vi "MRC Ds Comms Control Set Joystick Outputs.vi"(8 "error in (no error)":errorcluster, 10 "outputs":T1, 11 "stickIndex":i32) -> (0 "error out":errorcluster)   [LabVIEW 2026, in "MrcLib.lvlib"]
doc: "MRC_Status MRC_CALLCONV MRC_DsCommsControl_SetJoystickOutputs(int32_t stickIndex, const struct MRC_JoystickOutputs* outputs);"
uses:
  MrcLib.lvlib
  MrcLib.dll
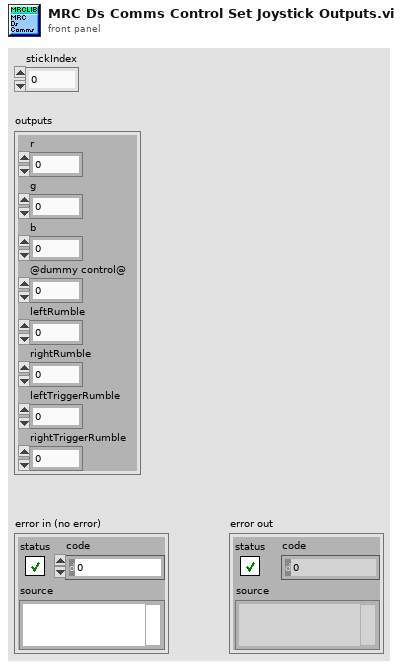
[diagram p1: front panel]
types:
  T1 = cluster{"r":u8, "g":u8, "b":u8, "@dummy control@":i8, "leftRumble":u16, "rightRumble":u16, "leftTriggerRumble":u16, "rightTriggerRumble":u16}
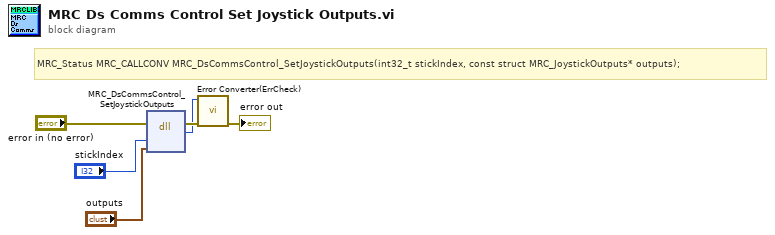
[diagram p0: block diagram]
diagram:
  # "MRC_Status MRC_CALLCONV MRC_DsCommsControl_SetJoystickOutputs(int32_t stickIndex, const struct MRC_JoystickOutputs* outputs);"
  n1 = dll-call lib="MrcLib.*" fn="MRC_DsCommsControl_SetJoystickOutputs"(error in="error in (no error)", "stickIndex"="stickIndex", "outputs"="outputs") -> (error out=w3:errorcluster, "return type"=w1:i32)  [unwired: 4 in, 1 out]
  n2 = call "Error Converter(ErrCheck).vi"("error in (no error)"=w3, "status"=w1) -> ("error out"=→"error out":errorcluster)  [unwired: 9 in]
